vi "Agilent VNA Format Data.vi"(6 "data format (f)\n(f: Form 3; t: Form 2)":bool, 8 "error in (no error)":errorcluster, 9 "Convert to dB? (f)":bool, 10 "Complex Data? (f:Single-Ended)":bool, 11 "Data String (\"\")":string) -> (0 "error out":errorcluster, 3 "Formatted Data":dbl[](array[numeric]))   [LabVIEW 2011]
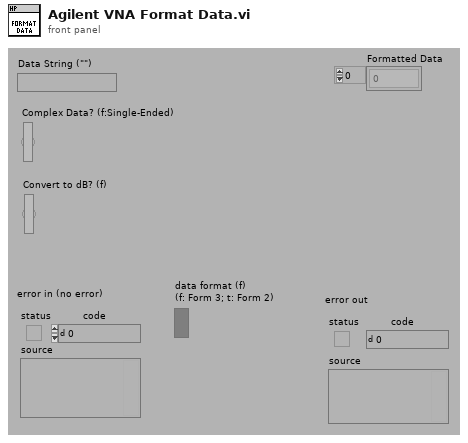
[diagram p1: front panel]
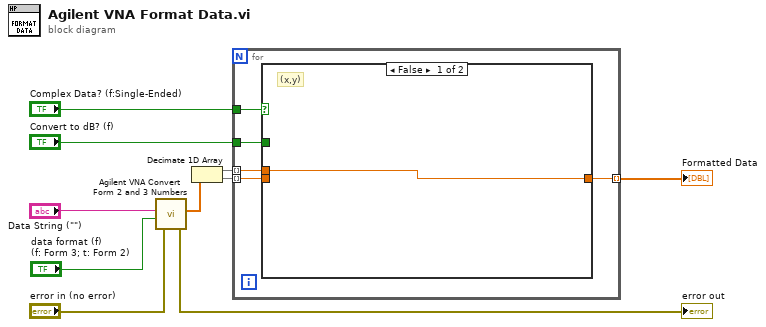
[diagram p0: block diagram]
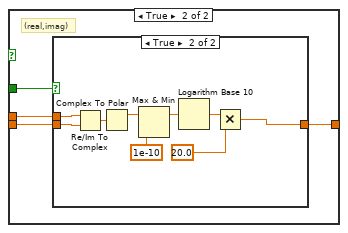
[diagram p2: hidden frame]
diagram:
  n1 = call "Agilent VNA Convert Form 2 and 3 Numbers.vi"("error in (no error)"="error in (no error)", "data format (f)\n(f: Form 3; t: Form 2)"="data format (f)\n(f: Form 3; t: Form 2)", "input string"="Data String (\"\")") -> ("error out"=→"error out":errorcluster, "Data"=w6:dbl[])  [unwired: 3 out]
  n2 = Decimate 1D Array(w6) -> (w10:dbl[], w9:dbl[])
  n3 = for {
    tunnel: w10 -> [w15] mode=indexing
    tunnel: w9 -> [w14] mode=indexing
    tunnel: "Complex Data? (f:Single-Ended)" -> [w13]
    tunnel: "Convert to dB? (f)" -> [w12]
    tunnel: [w11] -> w1 mode=indexing
    n4 = case shown="False" w13 {
      tunnel: w15 -> [w16 w19]
      tunnel: w14 -> [_ w18]
      tunnel: [w16 w17] -> w11
      tunnel: w12 -> [_ w20]
      frame False {
        # "(x,y)"
      }
      frame True {
        # "(real,imag)"
        n5 = case shown="True" w20 {
          tunnel: w19 -> [w21 w24]
          tunnel: w18 -> [_ w23]
          tunnel: [w21 w22] -> w17
          frame False {
          }
          frame True {
            n6 = Re/Im To Complex(1:w23, 2:w24) -> (0:w25:cdb)
            n7 = Complex To Polar(r * e^(i*theta)=w25) -> (r=w27:dbl)  [unwired: 1 out]
            n8 = Max & Min(x=w27, y=1e-10) -> (max(x,y)=w26:dbl)  [unwired: 1 out]
            n9 = Logarithm Base 10(1:w26) -> (0:w29:dbl)
            n10 = Multiply(x=w29, y=20.0) -> (x*y=w22:dbl)
          }
        }
      }
    }
  }
  "Formatted Data" <- w1
